vi "SQLite insert values.vi"(4 "Password":string, 5 "是否创建唯一键":bool, 6 "columns  INFO":string[](array[string]), 7 "数组":variant[][](array[variant]), 8 "错误输入（无错误）":errorcluster, 9 "columns外部输入":T1, 10 "database":string="database1.db", 11 "Tabe Name":string) -> (0 "错误输出":errorcluster)   [LabVIEW 2016, in "SQLite Lib.lvlib"]
uses:
  SQLite Lib.lvlib
  <userlib>/_LVST/sqlite_api/Core/Utils/SQLite_Pragma Cmd.ctl
  <userlib>/_LVST/sqlite_api/Core/Tables/SQLite_Create Table.vi
  <userlib>/_LVST/sqlite_api/Core/Tables/SQLite_List Columns.vi
  <userlib>/_LVST/sqlite_api/Core/Tables/SQLite_Add Column.vi
  <userlib>/_LVST/sqlite_api/Core/Insert/SQLite_Insert Table.vi
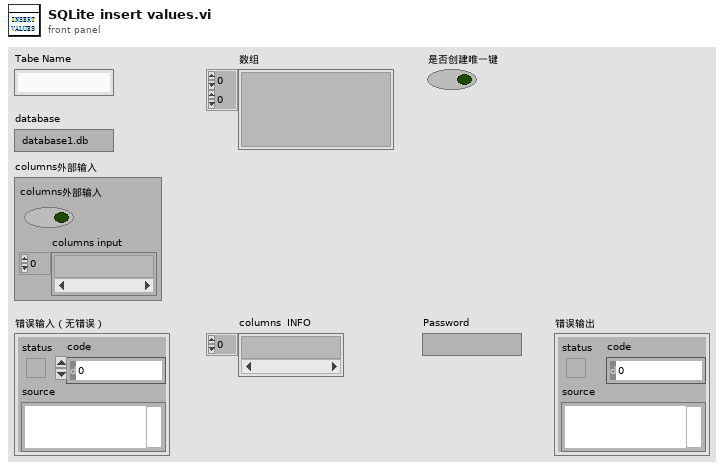
[diagram p1: front panel]
types:
  T1 = cluster{"columns外部输入":bool, "columns input":string[]}
  T2 = typedef "SQLite_Pragma Cmd.ctl" = u16
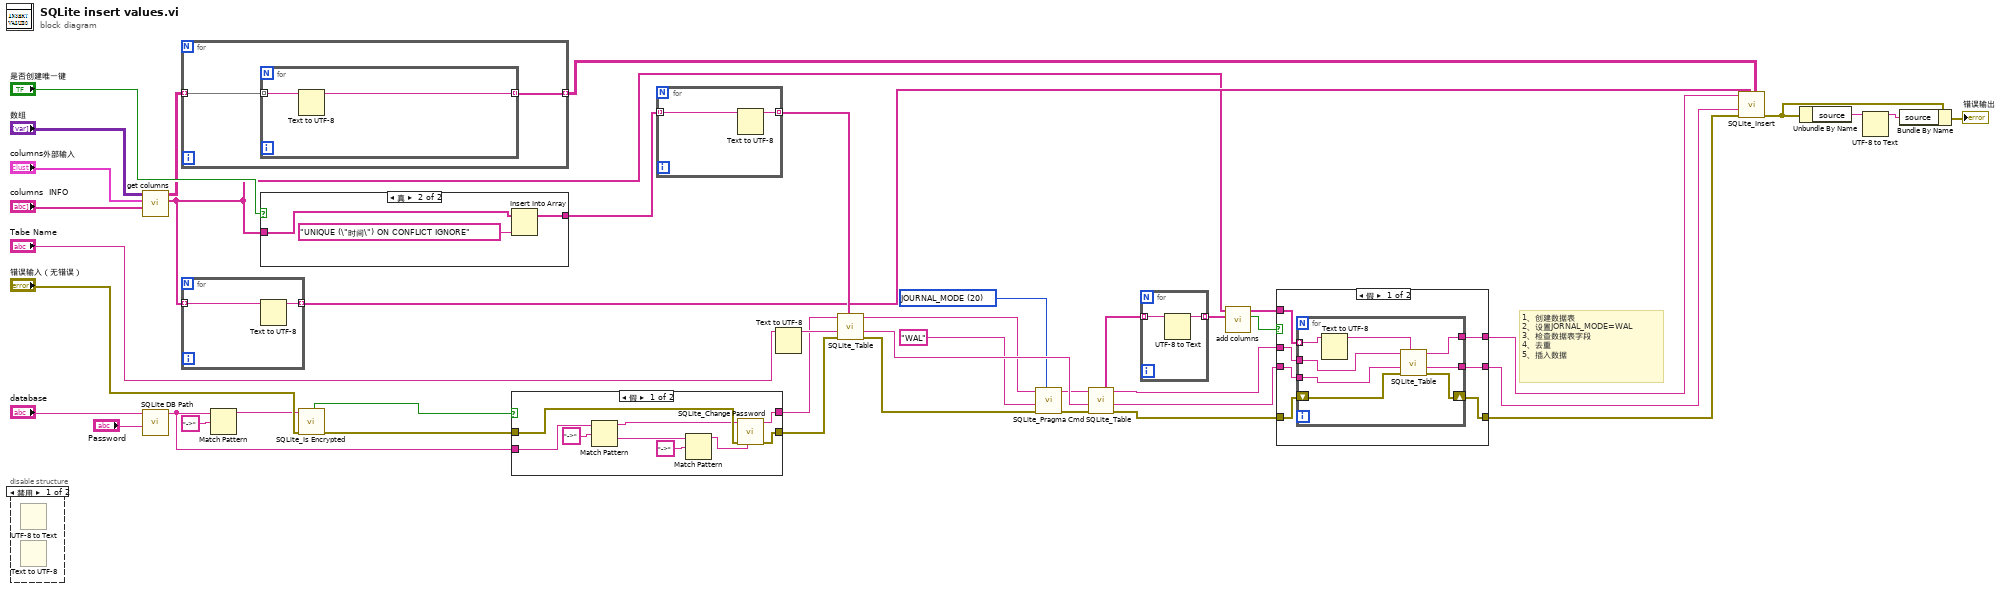
[diagram p0: block diagram]
diagram:
  w32 = T2 20 items=["AUTO_VACUUM", "AUTOMATIC_INDEX", "CACHE_SIZE", "CASE_SENSITIVE_LIKE", "COLLATION_LIST", "COMPILE_OPTIONS", "COUNT_CHANGES", "DATABASE_LIST", "DEFAULT_CACHE_SIZE", "EMPTY_RESULT_CALLBACKS", "ENCODING", "FOREIGN_KEY_LIST", "FOREIGN_KEYS", "FREELIST_COUNT", "FULL_COLUMN_NAMES", "FULLFSYNC", "INCREMENTAL_VACUUM", "INDEX_INFO", "INDEX_LIST", "INTEGRITY_CHECK", "JOURNAL_MODE", "JOURNAL_SIZE_LIMIT", "KEY", "LEGACY_FILE_FORMAT", "LOCKING_MODE", "MAX_PAGE_COUNT", "PAGE_COUNT", "PAGE_SIZE", "QUICK_CHECK", "READ_UNCOMMITTED", "REKEY", "RECURSIVE_TRIGGERS", "REVERSE_UNORDERED_SELECTS", "SCHEMA_VERSION", "SECURE_DELETE", "SHORT_COLUMN_NAMES", "SYNCHRONOUS", "TABLE_INFO", "TEMP_STORE", "TEMP_STORE_DIRECTORY", "USER_VERSION", "WAL_AUTOCHECKPOINT", "WAL_CHECKPOINT", "BUSY_TIMEOUT"] ("Cmd")
  # "1、创建数据表\n2、设置JORNAL_MODE=WAL\n3、检查数据表字段\n4、去重\n5、插入数据"
  n1 = disable-structure shown="禁用" {
    frame Disabled {
      n2 = UTF-8 to Text() -> ()  [unwired: 3 in, 2 out]
      n3 = Text to UTF-8() -> ()  [unwired: 3 in, 2 out]
    }
    frame Enabled {
    }
  }
  n4 = call "get columns.vi"("columns  INFO"="columns  INFO", "columns外部输入"="columns外部输入", "数组"="数组") -> ("columns output"=w10:string[], "data"=w13:string[][])  [unwired: 7 in]
  n5 = call "SQLite DB Path.vi"("Password"="Password", "database"="database") -> ("Path out"=w3:string)  [unwired: 9 in]
  n6 = for {
    tunnel: w13 -> [w45] mode=indexing
    tunnel: [w44] -> w12 mode=indexing
    n7 = for {
      tunnel: w45 -> [w47] mode=indexing
      tunnel: [w46] -> w44 mode=indexing
      n8 = Text to UTF-8(11:w47) -> (3:w46:string)  [unwired: 2 in, 1 out]
    }
  }
  n9 = for {
    tunnel: w10 -> [w49] mode=indexing
    tunnel: [w48] -> w14 mode=indexing
    n10 = Text to UTF-8(11:w49) -> (3:w48:string)  [unwired: 2 in, 1 out]
  }
  n11 = Match Pattern(string=w3, regular expression="->" ("正则表达式")) -> (before substring=w4:string)  [unwired: 1 in, 3 out]
  n12 = case shown="真" "是否创建唯一键" {
    tunnel: [w50 w53] -> w18
    tunnel: w10 -> [w50 w52]
    frame False {
    }
    frame True {
      n13 = Insert Into Array(array=w52, new element="UNIQUE (\"时间\") ON CONFLICT IGNORE" ("新元素/子数组")) -> (w53:string[])  [unwired: 1 in]
    }
  }
  n14 = call <userlib>:"SQLite_Is Encrypted.vi"("error in (no error)"="错误输入（无错误）", "Path"=w4) -> ("error out"=w8:errorcluster, "Encrypted?"=w7:bool)  [unwired: 6 in, 1 out]
  n15 = case shown="假" w7 {
    tunnel: w8 -> [w62 w63]
    tunnel: w3 -> [w55 w64]
    tunnel: [w54 w64] -> w6
    tunnel: [w61 w63] -> w5
    frame False {
      n16 = Match Pattern(string=w55, regular expression="->" ("正则表达式")) -> (before substring=w56:string, after substring=w59:string)  [unwired: 1 in, 2 out]
      n17 = Match Pattern(string=w59, regular expression="->" ("正则表达式")) -> (before substring=w57:string)  [unwired: 1 in, 3 out]
      n18 = call <userlib>:"SQLite_Change Password.vi"("New Password (Empty to remove)"=w57, "error in (no error)"=w62, "DB Path"=w56) -> ("error out"=w61:errorcluster, "Modified DB Path Out"=w54:string)  [unwired: 7 in]
    }
    frame True {
    }
  }
  n19 = for {
    tunnel: w18 -> [w66] mode=indexing
    tunnel: [w65] -> w17 mode=indexing
    n20 = Text to UTF-8(11:w66) -> (3:w65:string)  [unwired: 2 in, 1 out]
  }
  n21 = Text to UTF-8(11:"Tabe Name") -> (3:w19:string)  [unwired: 2 in, 1 out]
  n22 = call-poly <userlib>:"SQLite_Table.vi"("DB Path"=w6, "Table Name"=w19, "error in (no error)"=w5, "Columns"=w17) -> ("DB Path Out"=w30:string, "Table Name Out"=w33:string, "error out"=w28:errorcluster)  [unwired: 4 in]
  n23 = call <userlib>:"SQLite_Pragma Cmd.vi"("Cmd"=w32, "error in (no error)"=w28, "Value"="WAL" ("multi-line string"), "DB Path"=w30) -> ("error out"=w27:errorcluster, "DB Path Out"=w29:string)  [unwired: 3 in, 1 out]
  n24 = call-poly <userlib>:"SQLite_Table.vi"("DB Path"=w29, "Table Name"=w33, "error in (no error)"=w27) -> ("Columns"=w16:string[], "DB Path Out"=w40:string, "Table Name Out"=w39:string, "error out"=w38:errorcluster)  [unwired: 4 in]
  n25 = for {
    tunnel: w16 -> [w68] mode=indexing
    tunnel: [w67] -> w15 mode=indexing
    n26 = UTF-8 to Text(11:w68) -> (3:w67:string)  [unwired: 2 in, 1 out]
  }
  n27 = call "add columns.vi"("Old Col"=w15, "New Col"=w10) -> ("为空？"=w34:bool, "add col"=w41:string[])  [unwired: 8 in]
  n28 = case shown="假" w34 {
    tunnel: w41 -> [w75 _]
    tunnel: w40 -> [w74 w84]
    tunnel: w39 -> [w73 w85]
    tunnel: w38 -> [w69 w86]
    tunnel: [w72 w84] -> w37
    tunnel: [w71 w85] -> w36
    tunnel: [w70 w86] -> w35
    frame False {
      n29 = for {
        tunnel: w75 -> [w77] mode=indexing
        tunnel: w74 -> [w83]
        tunnel: w73 -> [w82]
        tunnel: [w81] -> w72
        tunnel: [w80] -> w71
        shift-right: [w79] -> w70
        shift-left: w69 -> [w78]
        n30 = Text to UTF-8(11:w77) -> (3:w76:string)  [unwired: 2 in, 1 out]
        n31 = call-poly <userlib>:"SQLite_Table.vi"("DB Path"=w83, "Table Name"=w82, "error in"=w78, "Field Declaration"=w76) -> ("DB Path Out"=w81:string, "Table Name Out"=w80:string, "error out"=w79:errorcluster)  [unwired: 4 in]
      }
    }
    frame True {
    }
  }
  n32 = call-poly <userlib>:"SQLite_Insert.vi"("Value Table"=w12, "Column"=w14, "error in"=w35, "Tabe Name"=w36, "DB Path"=w37) -> ("error out"=w26:errorcluster)  [unwired: 1 in, 3 out]
  n33 = Unbundle By Name(w26) -> ("source"=w25:string)
  n34 = UTF-8 to Text(11:w25) -> (3:w22:string)  [unwired: 2 in, 1 out]
  n35 = Bundle By Name(cluster=w26, "source"=w22) -> (→"错误输出":errorcluster)
